vi "文件操作.vi"() -> ()   [LabVIEW 2015]
panel:
  in  "文件路径":path
  in  "通道名输入（无标题）":string[](array[string])
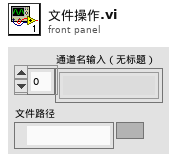
[diagram p1: front panel]
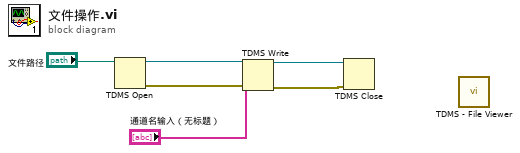
[diagram p0: block diagram]
diagram:
  n1 = TDMS Open(11:"文件路径") -> (0:w5:errorcluster, 3:w6:refnum<k34>)  [unwired: 6 in]
  n2 = TDMS Write(0:w6, 7:"通道名输入（无标题）", 11:w5) -> (4:w2:refnum<k34>, 15:w3:errorcluster)  [unwired: 3 in, 2 out]
  n3 = TDMS Close(8:w3, 11:w2) -> ()  [unwired: 2 out]
  n4 = call <vilib>:"TDMS - File Viewer.vi"() -> ()  [unwired: 6 in, 2 out]
